vi "NI VeriStand - Get Item Description.vi"(8 "error in (no error)":errorcluster, 11 "Item Ref in":T1 format="%.0x") -> (0 "error out":errorcluster, 2 "Description":string, 3 "Item Ref out":T1 format="%.0x", 4 "Found":bool)   [LabVIEW 2020, in "Custom Device Offline API.lvlib"]
uses:
  <vilib>/NI VeriStand/Custom Device Offline API/Custom Device Offline API.lvlib
  <vilib>/NI VeriStand/Custom Device API/Custom Device Item Ref.ctl
  NationalInstruments.VeriStand.SystemDefinitionAPI
  <vilib>/NI VeriStand/Custom Device API/Custom Device API.lvlib
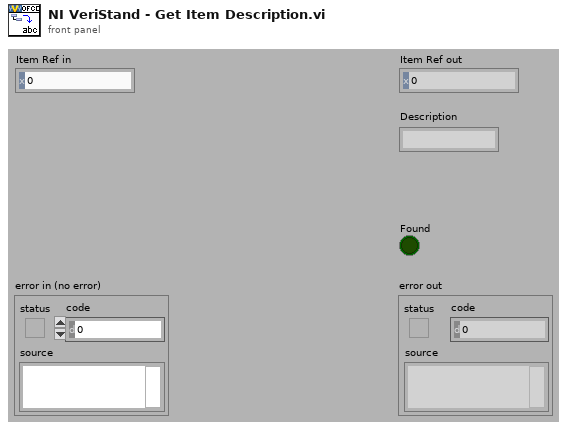
[diagram p1: front panel]
types:
  T1 = typedef "Custom Device API.lvlib/Custom Device Item Ref.ctl" = u64
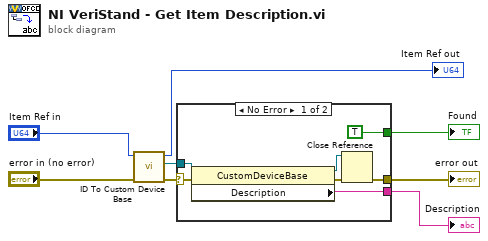
[diagram p0: block diagram]
diagram:
  n1 = call <vilib>:"ID To Custom Device Base.vi"("error in (no error)"="error in (no error)", "ID in"="Item Ref in") -> ("error out"=w7:errorcluster, "BaseNode"=w8:refnum<k24>, "ID out"=→"Item Ref out":u64)  [unwired: 7 in]
  n2 = case shown="No Error" w7 {
    selector: w7 -> [w14 w16]
    tunnel: w8 -> [w15 _]
    tunnel: [w11 w16] -> w3
    tunnel: [TRUE _] -> w2
    tunnel: [w9 _] -> w1
    frame No Error {
      n3 = property class="CustomDeviceBase"(reference=w15, error in=w14) -> (reference out=w13:refnum<k24>, error out=w12:errorcluster, "Description"=w9:string)
      n4 = Close Reference(reference=w13, error in (no error)=w12) -> (error out=w11:errorcluster)
    }
    frame Error {
    }
  }
  "Description" <- w1
  "error out" <- w3
  "Found" <- w2
